vi "Commutator_rxerr_parser.vi"(11 "String":string) -> (1 "Err no":i16, 2 "Err text":string, 3 "RX error":bool)   [LabVIEW 2011]
panel:
  in  "ErrComment_arr":string[](array[string])
  in  "Errno_arr":i16[](array[numeric])
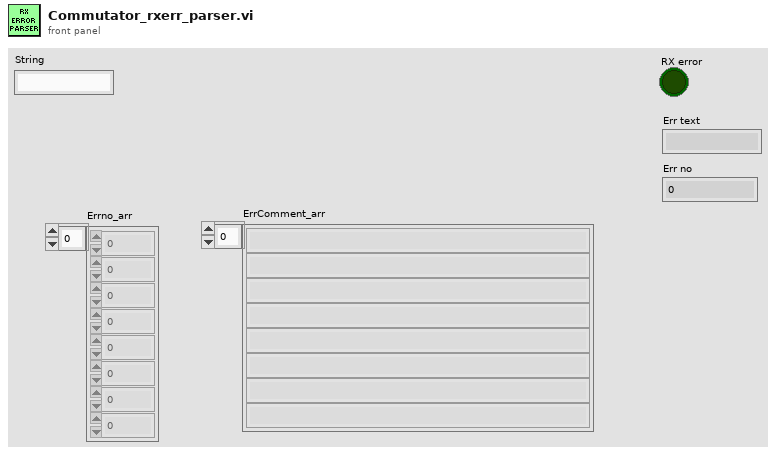
[diagram p1: front panel]
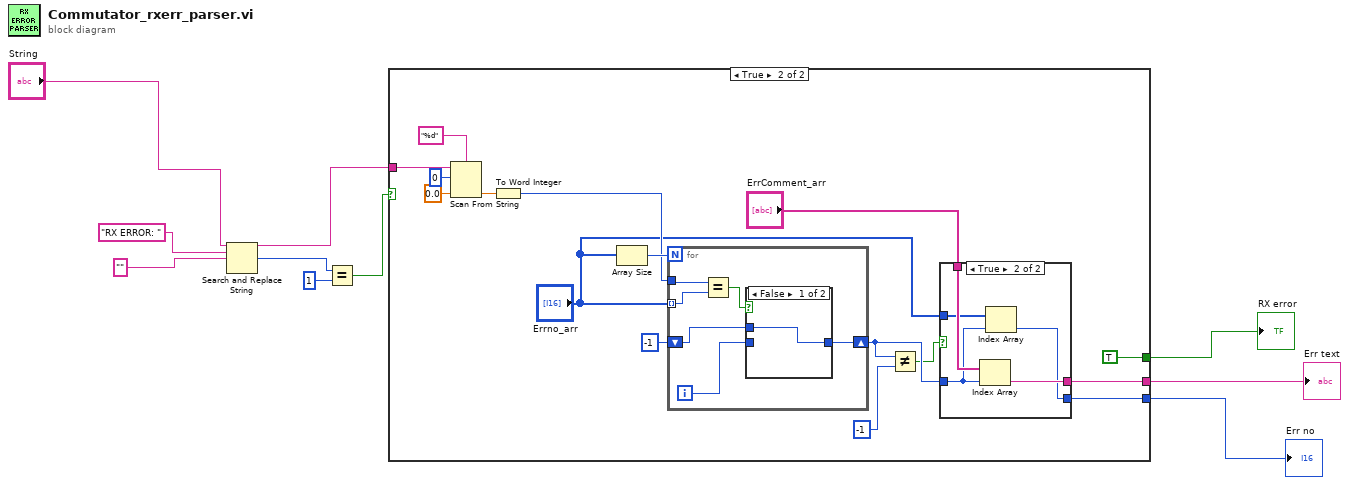
[diagram p0: block diagram]
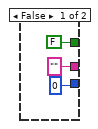
[diagram p2: hidden frame]
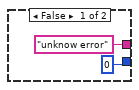
[diagram p3: hidden frame]
diagram:
  n1 = Search and Replace String(input string="String", search string="RX ERROR: ", replace string="" ("replace string (\"\")")) -> (result string=w5:string, number of replacements=w7:i32)  [unwired: 5 in, 2 out]
  n2 = Equal?(x=w7, y=1) -> (x = y?=w4:bool)
  n3 = case shown="True" w4 {
    tunnel: w5 -> [_ w29]
    tunnel: ["" ("String 2") w17] -> w2
    tunnel: [FALSE TRUE] -> w3
    tunnel: [i16 0 ("Numeric") w14] -> w1
    frame False {
    }
    frame True {
      n4 = Scan From String(format string="%d", input string=w29, initial scan location=u32 0, default 1=0.0 ("default value 1")) -> (output 1=w25:dbl)  [unwired: 1 in, 3 out]
      n5 = To Word Integer(number=w25) -> (16bit integer=w18:i16)
      n6 = Array Size(array="Errno_arr") -> (size(s)=w21:i32)
      n7 = for {
        N: w21 -> [_]
        tunnel: "Errno_arr" -> [w41] mode=indexing
        tunnel: w18 -> [w42]
        shift-right: [w39] -> w24
        shift-left: -1 -> [w37]
        i -> [w38]
        n8 = Equal?(x=w42, y=w41) -> (x = y?=w40:bool)
        n9 = case shown="False" w40 {
          tunnel: [w43 w44] -> w39
          tunnel: w38 -> [_ w44]
          tunnel: w37 -> [w43 _]
          frame False {
          }
          frame True {
          }
        }
      }
      n10 = Not Equal?(x=w24, y=-1) -> (x != y?=w22:bool)
      n11 = case shown="True" w22 {
        tunnel: "ErrComment_arr" -> [_ w36]
        tunnel: w24 -> [_ w33]
        tunnel: ["unknow error" ("String 2") w35] -> w17
        tunnel: [i16 0 ("Numeric") w32] -> w14
        tunnel: "Errno_arr" -> [_ w34]
        frame False {
        }
        frame True {
          n12 = Index Array(array=w36, index=w33) -> (element=w35:string)
          n13 = Index Array(array=w34, index=w33) -> (element=w32:i16)
        }
      }
    }
  }
  "RX error" <- w3
  "Err text" <- w2
  "Err no" <- w1
